vi "Set Results.vi"(8 "error in (no error)":errorcluster, 10 "Sequence Context":refnum<k7>, 11 "PostUUT in":refnum<class "PostUUT.lvclass">) -> (0 "error out":errorcluster, 3 "PostUUT out":refnum<class "PostUUT.lvclass">)   [LabVIEW 2021, in "OPC UA.lvlib" / "PostUUT.lvclass"]
uses:
  PostUUT.lvclass
  PostUUT.lvclass/PostUUT.ctl
  <vilib>/addons/TestStand/_TSUtility.llb/TestStand - Get Property Value (Number {Signed 32-bit Integer}).vi
  <vilib>/addons/TestStand/_TSUtility.llb/TestStand - Get Property Value (String).vi
  <vilib>/addons/TestStand/_TSUtility.llb/TestStand - Set Property Value (Boolean).vi
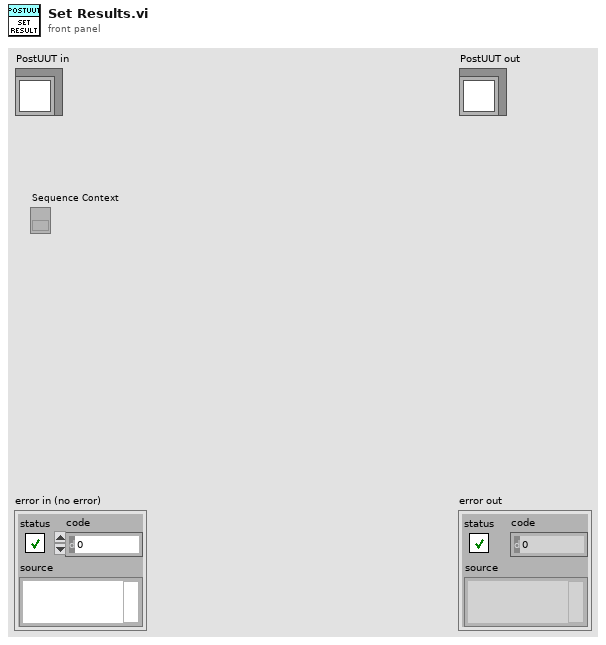
[diagram p1: front panel]
types:
  T1 = cluster{"Result":i32, "Result Status":string, "Elapsed Time":i32}
  T2 = typedef "LVDateTimeRec.ctl" = cluster{"fractional second":dbl, "second":i32, "minute":i32, "hour":i32, "day of month":i32, "month":i32, "year":i32, "day of week":i32, "day of year":i32, "DST":i32}
  T3 = cluster{"fractional second":i32, "second":i32, "minute":i32, "hour":i32, "day of month":i32, "month":i32, "year":i32, "day of week":i32, "day of year":i32, "DST":i32}
  T4 = typedef "PostUUT.lvclass/Tx PostUUT.ctl" = cluster{"ResultsReady":bool, "Results":u32, "ElapsedTime":i32, "TimeCompleted":i32[], "Fault":bool, "Timeout":bool}
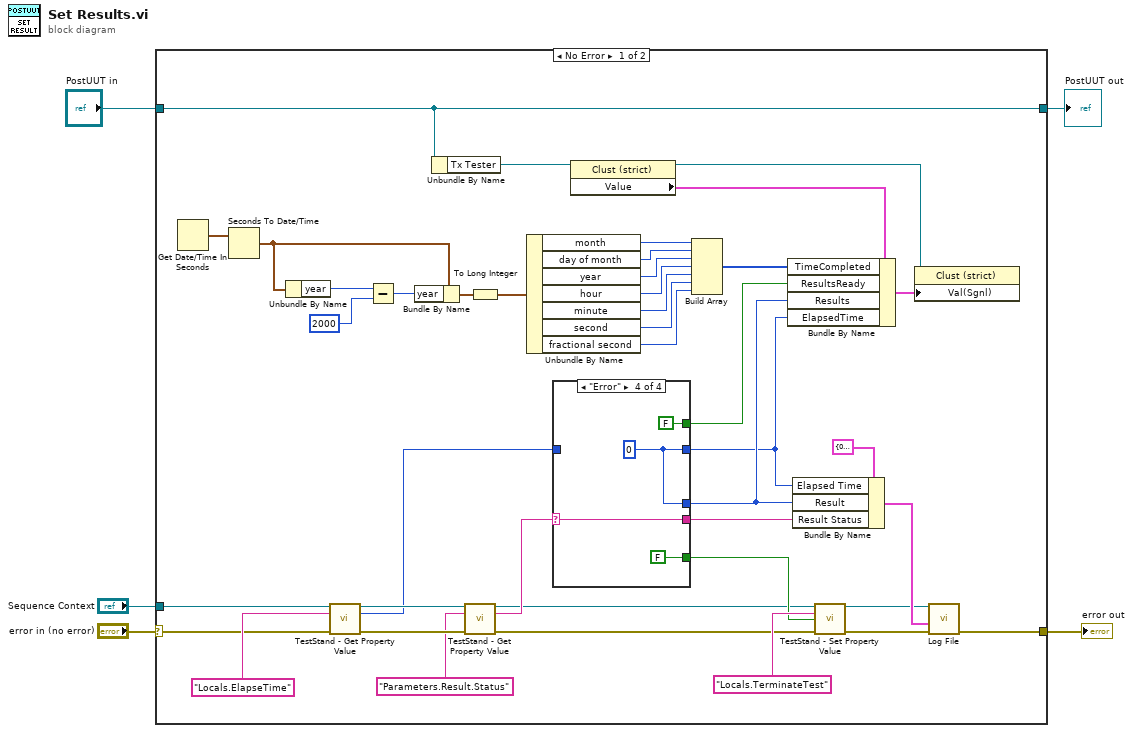
[diagram p0: block diagram]
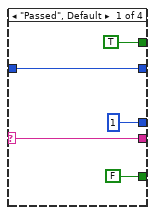
[diagram p2: hidden frame]
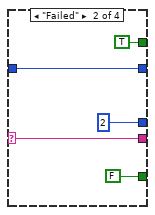
[diagram p3: hidden frame]
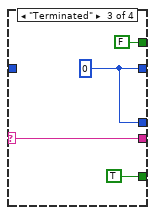
[diagram p4: hidden frame]
diagram:
  n1 = case shown="No Error" "error in (no error)" {
    selector: "error in (no error)" -> [w9 w66]
    tunnel: [w12 w66] -> w4
    tunnel: [w29 w65] -> w2
    tunnel: "PostUUT in" -> [w29 w65]
    tunnel: "Sequence Context" -> [w10 _]
    frame No Error {
      n2 = Get Date/Time In Seconds() -> (seconds since 1Jan1904=w44:timestamp)
      n3 = Seconds To Date/Time(time stamp (now)=w44) -> (date time rec=w33:T2)  [unwired: 1 in]
      n4 = Unbundle By Name(w33) -> ("year"=w31:i32)
      n5 = call-poly <vilib>:"TestStand - Get Property Value.vi"("Sequence Context In"=w10, "Lookup String"="Locals.ElapseTime", "error in (no error)"=w9) -> ("Sequence Context Out"=w24:refnum<k7>, "Value"=w7:i32, "error out"=w27:errorcluster)  [unwired: 10 in]
      n6 = Subtract(x=w31, y=2000) -> (x-y=w34:i32)
      n7 = Bundle By Name(cluster=w33, "year"=w34) -> (w35:T2)
      n8 = Unbundle By Name(w29) -> ("Tx Tester"=w46:refnum<vi>)
      n9 = call-poly <vilib>:"TestStand - Get Property Value.vi"("Sequence Context In"=w24, "Lookup String"="Parameters.Result.Status", "error in (no error)"=w27) -> ("Sequence Context Out"=w19:refnum<k7>, "Value"=w23:string, "error out"=w21:errorcluster)  [unwired: 10 in]
      n10 = To Long Integer(number=w35) -> (32bit integer=w36:T3)
      n11 = Unbundle By Name(w36) -> ("month"=w37:i32, "day of month"=w38:i32, "year"=w39:i32, "hour"=w40:i32, "minute"=w41:i32, "second"=w42:i32, "fractional second"=w43:i32)
      n12 = case shown="\"Error\"" w23 {
        selector: w23 -> [w50 w55 w60 w64]
        tunnel: [1 2 w57 w61] -> w17
        tunnel: [w50 w55 w60 w64] -> w16
        tunnel: [FALSE ("ResultsReady") FALSE ("ResultsReady") TRUE ("ResultsReady") FALSE ("ResultsReady")] -> w20
        tunnel: [TRUE ("ResultsReady") TRUE ("ResultsReady") FALSE ("ResultsReady") FALSE ("ResultsReady")] -> w8
        tunnel: w7 -> [w47 w52 _ _]
        tunnel: [w47 w52 w57 w61] -> w6
        frame "Passed", Default {
        }
        frame "Failed" {
        }
        frame "Terminated" {
          w57 = 0 ("Value")
        }
        frame "Error" {
          w61 = 0 ("Value")
        }
      }
      n13 = property class="Clust (strict)"(reference=w46) -> (reference out=w28:refnum<vi>, "Value"=w30:T4)  [unwired: 1 in, 1 out]
      n14 = Build Array(w37, w38, w39, w40, w41, w42, w43) -> (w45:i32[])
      n15 = Bundle By Name(cluster=w30, "TimeCompleted"=w45, "ResultsReady"=w8, "Results"=w17, "ElapsedTime"=w6) -> (w11:T4)
      n16 = Bundle By Name(cluster=T1 {"Result"=0, "Result Status"="", "Elapsed Time"=0}, "Elapsed Time"=w6, "Result"=w17, "Result Status"=w16) -> (w14:T1)
      n17 = call-poly <vilib>:"TestStand - Set Property Value.vi"("Sequence Context In"=w19, "Lookup String"="Locals.TerminateTest", "New Value"=w20, "error in (no error)"=w21) -> ("Sequence Context Out"=w13:refnum<k7>, "error out"=w15:errorcluster)  [unwired: 10 in]
      n18 = property class="Clust (strict)"(reference=w28, "Val(Sgnl)"=w11) -> ()  [unwired: 1 in, 2 out]
      n19 = call "Log File.vi"("error in"=w15, "Test Result"=w14, "Sequence Context"=w13) -> ("error out"=w12:errorcluster)  [unwired: 8 in]
    }
    frame Error {
    }
  }
  "error out" <- w4
  "PostUUT out" <- w2
